vi "Upgrade Addon to Latest Version.vi"(8 "error in (no error)":errorcluster, 11 "Device Item Ref in in":T1 format="%.0x") -> (0 "error out":errorcluster, 3 "Device Item Ref out":T1 format="%.0x")   [LabVIEW 2019, in "FPGA Addon Shared.lvlib"]
uses:
  FPGA Addon Shared.lvlib
  FG Action.ctl
  Constants.vi
  Data Type.ctl
  Register Information.ctl
  <vilib>/NI/NI VeriStand Advanced SysDef API/SysDef API/Advanced System Definition.lvlib
  <vilib>/NI/NI VeriStand Advanced SysDef API/_SubVIs/SysDef.Search.GUID.vi
  <vilib>/NI/NI VeriStand Advanced SysDef API/_SubVIs/SysDef.Property.Get.Variant.vi
  <vilib>/rvi/ClientSDK/Core/ModuleGeneration/CommunicationInterfaceUtility/niFpgaDmaChannelImplementation.ctl
  <vilib>/rvi/DataTransferAndStorage/Container/Common/niFpgaDataTypeControl.ctl
  <vilib>/rvi/FIFO/Fifo_Types/Fifo_DMA_Config.ctl
  DMA Information.ctl
  NationalInstruments.VeriStand.SystemDefinitionAPI
  <vilib>/NI VeriStand/Custom Device API/Custom Device Item Ref.ctl
  <vilib>/NI VeriStand/Custom Device API/Custom Device API.lvlib
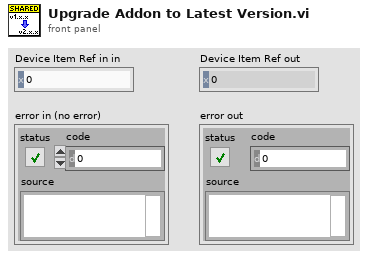
[diagram p1: front panel]
types:
  T1 = typedef "Custom Device API.lvlib/Custom Device Item Ref.ctl" = u64
  T2 = typedef "FPGA Addon Shared.lvlib/FG Action.ctl" = enum8{"GET", "SET"}
  T3 = typedef "FPGA Addon Shared.lvlib/Register Information.ctl" = cluster{"Name":string, "Data Type":T4, "Default Value":variant}
  T4 = typedef "FPGA Addon Shared.lvlib/Data Type.ctl" = enum8{"<Null>", "I8", "I16", "I32", "I64", "U8", "U16", "U32", "U64", "SGL", "Boolean", "Analog PWM In Settings", "Analog PWM In", "Digital PWM In Settings", "Digital PWM In", "Digital PWM Out", "Sine Out", "FXP+/-24.5", "FXP+/-16.5", "FXP+/-32.8", "FXP+/-64.32", "FXP+/-16.7", "FXP+/-20.5", "FXP+/-27.5", "FXP+/-32.16", "FXP +16.3", "FXP +18.3", "Digital Static In", "Digital Static Out", "Digital Static In Settings", "Digital WSS Out", "Quad Encoder Settings", "Quad Encoder In"}
  T5 = typedef "FPGA Addon Shared.lvlib/DMA Information.ctl" = cluster{"Name":string, "Data Type":T4}
  T6 = cluster{"Name":string, "Data Type":enum8{"<Null>", "I8", "I16", "I32", "I64", "U8", "U16", "U32", "U64", "SGL", "DBL", "EXT", "CSG", "CDB", "CXT", "0x0F", "0x10", "0x11", "0x12", "0x13", "0x14", "Enum U8", "Enum U16", "Enum U32", "Enum U64", "SGL PQ", "DBL PQ", "EXT PQ", "CSG PQ", "CDB PQ", "CXT PQ", "0x1F", "0x20", "Boolean", "0x22", "0x23", "0x24", "0x25", "0x26", "0x27", "0x28", "0x29", "0x2A", "0x2B", "0x2C", "0x2D", "0x2E", "0x2F", "String", "0x31", "Path", "Pict", "0x34", "0x35", "0x36", "DAQ", "0x38", "0x39", "0x3A", "0x3B", "0x3C", "0x3D", "0x3E", "0x3F", "Array", "0x41", "0x42", "0x43", "0x44", "0x45", "0x46", "0x47", "0x48", "0x49", "0x4A", "0x4B", "0x4C", "0x4D", "0x4E", "0x4F", "Cluster", "0x51", "0x52", "Variant", "Waveform", "0x55", "0x56", "0x57", "0x58", "0x59", "0x5A", "0x5B", "0x5C", "0x5D", "0x5E", "0x5F", "0x60", "0x61", "0x62", "0x63", "0x64", "0x65", "0x66", "0x67", "0x68", "0x69", "0x6A", "0x6B", "0x6C", "0x6D", "0x6E", "0x6F", "Refnum"}, "Default Value":dbl}[]
  T7 = enum8{"<Null>", "I8", "I16", "I32", "I64", "U8", "U16", "U32", "U64", "SGL", "DBL", "EXT", "CSG", "CDB", "CXT", "0x0F", "0x10", "0x11", "0x12", "0x13", "0x14", "Enum U8", "Enum U16", "Enum U32", "Enum U64", "SGL PQ", "DBL PQ", "EXT PQ", "CSG PQ", "CDB PQ", "CXT PQ", "0x1F", "0x20", "Boolean", "0x22", "0x23", "0x24", "0x25", "0x26", "0x27", "0x28", "0x29", "0x2A", "0x2B", "0x2C", "0x2D", "0x2E", "0x2F", "String", "0x31", "Path", "Pict", "0x34", "0x35", "0x36", "DAQ", "0x38", "0x39", "0x3A", "0x3B", "0x3C", "0x3D", "0x3E", "0x3F", "Array", "0x41", "0x42", "0x43", "0x44", "0x45", "0x46", "0x47", "0x48", "0x49", "0x4A", "0x4B", "0x4C", "0x4D", "0x4E", "0x4F", "Cluster", "0x51", "0x52", "Variant", "Waveform", "0x55", "0x56", "0x57", "0x58", "0x59", "0x5A", "0x5B", "0x5C", "0x5D", "0x5E", "0x5F", "0x60", "0x61", "0x62", "0x63", "0x64", "0x65", "0x66", "0x67", "0x68", "0x69", "0x6A", "0x6B", "0x6C", "0x6D", "0x6E", "0x6F", "Refnum"}
  T8 = typedef "Fifo_DMA_Config.ctl" = cluster{"Name":string, "Depth":u32, "Write? (Deprecated:Use Implementation)":bool, "Physical Channel":u32, "Base Address":u32, "Data Width":u32, "Data Type":T9, "FXP Properties":variant, "Write Window Address":u32, "Implementation":T10, "Control Set":u32}
  T9 = typedef "niFpgaDataTypeControl.ctl" = enum32{"Boolean", "I8", "I16", "I32", "I64", "U8", "U16", "U32", "U64", "FXP", "CustomControl", "SGL"}
  T10 = typedef "niFpgaDmaChannelImplementation.ctl" = enum16{"niFpgaTargetToHost", "niFpgaHostToTarget", "niFpgaPeerToPeerWriter", "niFpgaPeerToPeerReader", "niCoreTargetToHost", "niCoreHostToTarget"}
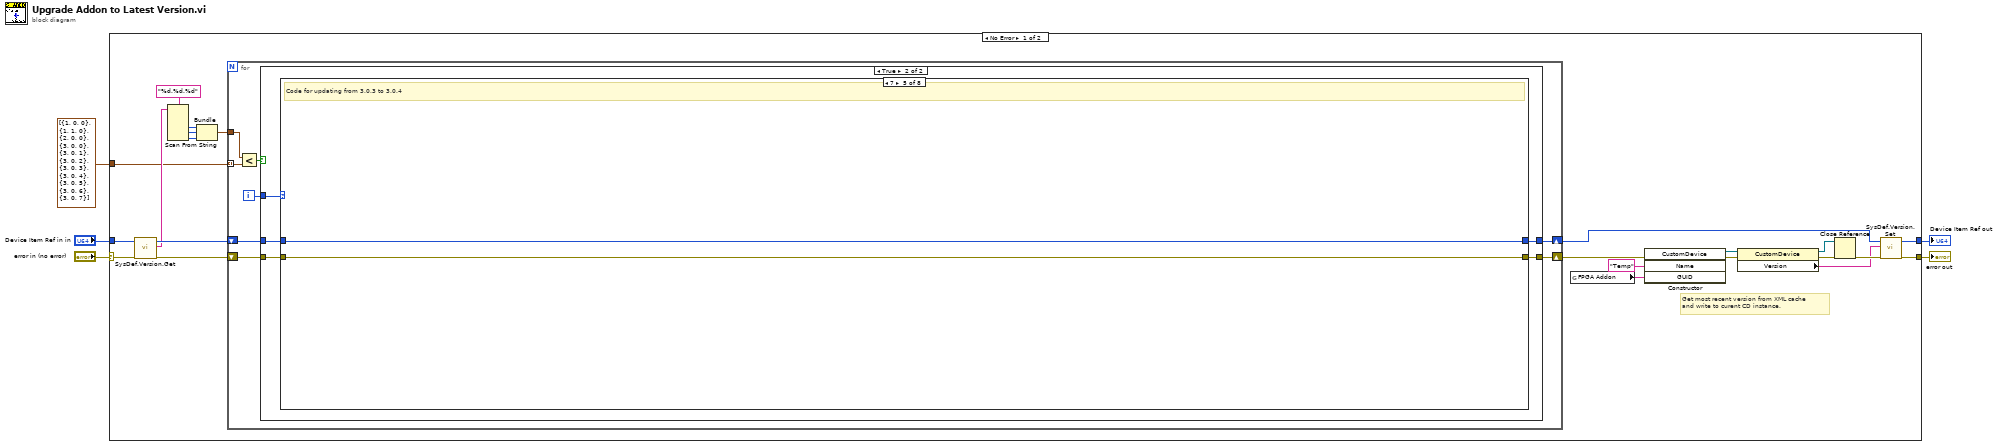
[diagram p0: block diagram]
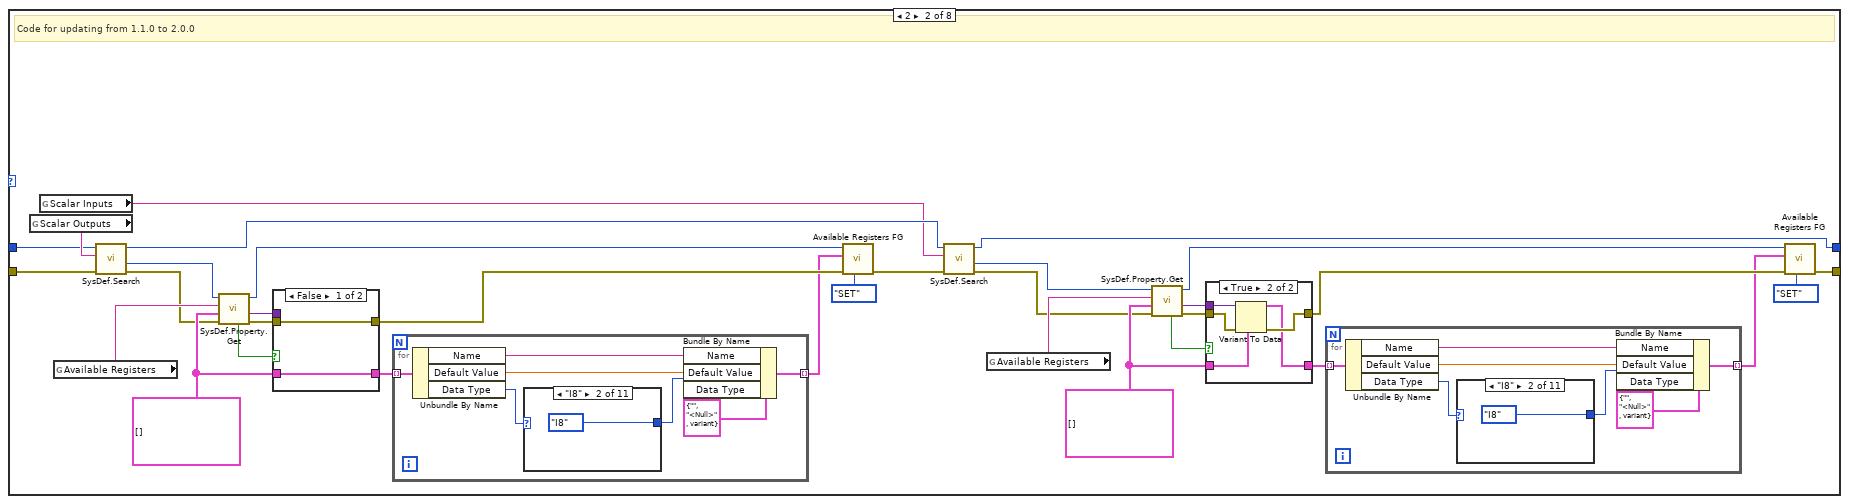
[diagram p4: hidden frame]
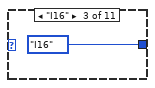
[diagram p6: hidden frame]
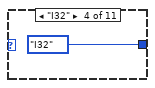
[diagram p7: hidden frame]
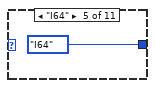
[diagram p8: hidden frame]
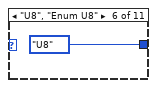
[diagram p9: hidden frame]
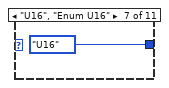
[diagram p10: hidden frame]
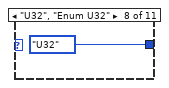
[diagram p11: hidden frame]
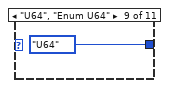
[diagram p12: hidden frame]
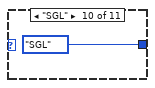
[diagram p13: hidden frame]
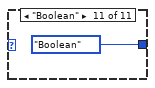
[diagram p14: hidden frame]
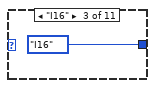
[diagram p17: hidden frame]
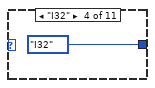
[diagram p18: hidden frame]
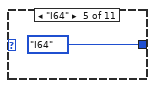
[diagram p19: hidden frame]
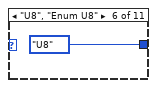
[diagram p20: hidden frame]
diagram:
  n1 = case shown="No Error" "error in (no error)" {
    selector: "error in (no error)" -> [w12 w193]
    tunnel: [w22 w193] -> w4
    tunnel: "Device Item Ref in in" -> [w11 w192]
    tunnel: [w21 w192] -> w5
    tunnel: cluster{i32, i32, i32}[] [{1, 0, 0}, {1, 1, 0}, {2, 0, 0}, {3, 0, 0}, {3, 0, 1}, {3, 0, 2}, {3, 0, 3}, {3, 0, 4}, {3, 0, 5}, {3, 0, 6}, {3, 0, 7}] -> [w6 _]
    frame No Error {
      # "Get most recent version from XML cache\nand write to curent CD instance."
      n2 = call <vilib>:"SysDef.Version.Get.vi"("error in (no error)"=w12, "nodeID"=w11) -> ("error out"=w9:errorcluster, "Version"=w8:string, "nodeID out"=w10:u64)  [unwired: 7 in]
      n3 = Scan From String(format string="%d.%d.%d", input string=w8) -> (output 1=w15:i32, output 2=w14:i32, output 3=w16:i32)  [unwired: 5 in, 3 out]
      n4 = Bundle(w15, w14, w16) -> (w7:cluster{i32, i32, i32})  [unwired: 1 in]
      n5 = for {
        shift-right: [w36] -> w19
        shift-left: w9 -> [w29]
        shift-right: [w35] -> w20
        shift-left: w10 -> [w30]
        tunnel: w7 -> [w33]
        tunnel: w6 -> [w31] mode=indexing
        i -> [w34]
        n6 = Less?(x=w33, y=w31) -> (x < y?=w32:bool)
        n7 = case shown="True" w32 {
          tunnel: w29 -> [w38 w43]
          tunnel: [w38 w42] -> w36
          tunnel: w30 -> [w37 w39]
          tunnel: [w37 w40] -> w35
          tunnel: w34 -> [_ w41]
          frame False {
          }
          frame True {
            n8 = case shown="7" w41 {
              tunnel: w43 -> [w45 w71 w151 w183 w185 w187 w189 w191]
              tunnel: [w45 w46 w127 w183 w185 w187 w189 w191] -> w42
              tunnel: [w44 w47 w128 w182 w184 w186 w188 w190] -> w40
              tunnel: w39 -> [w44 w70 w150 w182 w184 w186 w188 w190]
              frame Default {
              }
              frame 2 {
                w54 = T6 [] ("Available Registers 2")
                w65 = T6 [] ("Available Registers 2")
                # "Code for updating from 1.1.0 to 2.0.0"
                n9 = global read "Constants.vi" "Scalar Outputs"() -> (w76:string)
                n10 = global read "Constants.vi" "Scalar Inputs"() -> (w72:string)
                n11 = global read "Constants.vi" "Available Registers"() -> (w66:string)
                n12 = call-poly <vilib>:"SysDef.Search.vi"("error in (no error)"=w71, "GUID"=w76, "nodeID"=w70) -> ("error out"=w62:errorcluster, "Value out"=w64:u64, "nodeID out"=w73:u64)  [unwired: 5 in, 1 out]
                n13 = call-poly <vilib>:"SysDef.Property.Get.vi"("error in (no error)"=w62, "Value"=w65, "Property Name"=w66, "nodeID"=w64) -> ("error out"=w68:errorcluster, "Value"=w67:variant, "nodeID out"=w63:u64, "Found?"=w69:bool)  [unwired: 4 in]
                n14 = case shown="False" w69 {
                  tunnel: w67 -> [_ w125]
                  tunnel: w65 -> [w119 w124]
                  tunnel: w68 -> [w120 w123]
                  tunnel: [w120 w122] -> w61
                  tunnel: [w119 w121] -> w60
                  frame False {
                  }
                  frame True {
                    n15 = Variant To Data(error in=w123, type=w124, Variant=w125) -> (data=w121:T6, error out=w122:errorcluster)
                  }
                }
                n16 = for {
                  tunnel: w60 -> [w108] mode=indexing
                  tunnel: [w104] -> w59 mode=indexing
                  n17 = Unbundle By Name(w108) -> ("Name"=w107:string, "Default Value"=w106:dbl, "Data Type"=w103:T7)
                  n18 = case shown="\"I8\"" w103 {
                    tunnel: [_ Data_Type."I8" ("Data Type") Data_Type."I16" ("Data Type") Data_Type."I32" ("Data Type") Data_Type."I64" ("Data Type") Data_Type."U8" ("Data Type") Data_Type."U16" ("Data Type") Data_Type."U32" ("Data Type") Data_Type."U64" ("Data Type") Data_Type."SGL" ("Data Type") Data_Type."Boolean" ("Data Type")] -> w102
                    frame Default {
                    }
                    frame "I8" {
                    }
                    frame "I16" {
                    }
                    frame "I32" {
                    }
                    frame "I64" {
                    }
                    frame "U8", "Enum U8" {
                    }
                    frame "U16", "Enum U16" {
                    }
                    frame "U32", "Enum U32" {
                    }
                    frame "U64", "Enum U64" {
                    }
                    frame "SGL" {
                    }
                    frame "Boolean" {
                    }
                  }
                  n19 = Bundle By Name(cluster=T3 {"Name"="", "Data Type"=enum."<Null>", "Default Value"=variant(refnum<class> refnum)}, "Name"=w107, "Default Value"=w106, "Data Type"=w102) -> (w104:T3)
                }
                n20 = call "Available Registers FG.vi"("Action"=FG_Action."SET", "error in (no error)"=w61, "Available Registers"=w59, "Item Ref"=w63) -> ("error out"=w74:errorcluster)  [unwired: 5 in, 2 out]
                n21 = call-poly <vilib>:"SysDef.Search.vi"("error in (no error)"=w74, "GUID"=w72, "nodeID"=w73) -> ("error out"=w52:errorcluster, "Value out"=w49:u64, "nodeID out"=w47:u64)  [unwired: 5 in, 1 out]
                n22 = global read "Constants.vi" "Available Registers"() -> (w55:string)
                n23 = call-poly <vilib>:"SysDef.Property.Get.vi"("error in (no error)"=w52, "Value"=w54, "Property Name"=w55, "nodeID"=w49) -> ("error out"=w57:errorcluster, "Value"=w56:variant, "nodeID out"=w48:u64, "Found?"=w58:bool)  [unwired: 4 in]
                n24 = case shown="True" w58 {
                  tunnel: w56 -> [_ w101]
                  tunnel: w54 -> [w95 w100]
                  tunnel: w57 -> [w96 w99]
                  tunnel: [w96 w98] -> w51
                  tunnel: [w95 w97] -> w53
                  frame False {
                  }
                  frame True {
                    n25 = Variant To Data(error in=w99, type=w100, Variant=w101) -> (data=w97:T6, error out=w98:errorcluster)
                  }
                }
                n26 = for {
                  tunnel: w53 -> [w84] mode=indexing
                  tunnel: [w80] -> w50 mode=indexing
                  n27 = Unbundle By Name(w84) -> ("Name"=w83:string, "Default Value"=w82:dbl, "Data Type"=w79:T7)
                  n28 = case shown="\"I8\"" w79 {
                    tunnel: [_ Data_Type."I8" ("Data Type") Data_Type."I16" ("Data Type") Data_Type."I32" ("Data Type") Data_Type."I64" ("Data Type") Data_Type."U8" ("Data Type") Data_Type."U16" ("Data Type") Data_Type."U32" ("Data Type") Data_Type."U64" ("Data Type") Data_Type."SGL" ("Data Type") Data_Type."Boolean" ("Data Type")] -> w78
                    frame Default {
                    }
                    frame "I8" {
                    }
                    frame "I16" {
                    }
                    frame "I32" {
                    }
                    frame "I64" {
                    }
                    frame "U8", "Enum U8" {
                    }
                    frame "U16", "Enum U16" {
                    }
                    frame "U32", "Enum U32" {
                    }
                    frame "U64", "Enum U64" {
                    }
                    frame "SGL" {
                    }
                    frame "Boolean" {
                    }
                  }
                  n29 = Bundle By Name(cluster=T3 {"Name"="", "Data Type"=enum."<Null>", "Default Value"=variant(refnum<class> refnum)}, "Name"=w83, "Default Value"=w82, "Data Type"=w78) -> (w80:T3)
                }
                n30 = call "Available Registers FG.vi"("Action"=FG_Action."SET", "error in (no error)"=w51, "Available Registers"=w50, "Item Ref"=w48) -> ("error out"=w46:errorcluster)  [unwired: 5 in, 2 out]
              }
              frame 5 {
                w126 = T8[] [] ("Available Registers 2")
                w135 = T8[] [] ("Available Registers 2")
                # "Code for updating from 3.0.1 to 3.0.2"
                n31 = global read "Constants.vi" "Waveform Outputs"() -> (w152:string)
                n32 = global read "Constants.vi" "Waveform Inputs"() -> (w156:string)
                n33 = global read "Constants.vi" "Available DMA"() -> (w146:string)
                n34 = call-poly <vilib>:"SysDef.Search.vi"("error in (no error)"=w151, "GUID"=w156, "nodeID"=w150) -> ("error out"=w143:errorcluster, "Value out"=w145:u64, "nodeID out"=w153:u64)  [unwired: 5 in, 1 out]
                n35 = call-poly <vilib>:"SysDef.Property.Get.vi"("error in (no error)"=w143, "Value"=w126, "Property Name"=w146, "nodeID"=w145) -> ("error out"=w148:errorcluster, "Value"=w147:variant, "nodeID out"=w144:u64, "Found?"=w149:bool)  [unwired: 4 in]
                n36 = case shown="False" w149 {
                  tunnel: w147 -> [_ w181]
                  tunnel: w126 -> [w175 w180]
                  tunnel: w148 -> [w176 w179]
                  tunnel: [w176 w178] -> w142
                  tunnel: [w175 w177] -> w141
                  frame False {
                  }
                  frame True {
                    n37 = Variant To Data(error in=w179, type=w180, Variant=w181) -> (data=w177:T8[], error out=w178:errorcluster)
                  }
                }
                n38 = for {
                  tunnel: w141 -> [w174] mode=indexing
                  tunnel: [w172] -> w140 mode=indexing
                  n39 = Unbundle By Name(w174) -> ("Name"=w173:string)
                  n40 = Bundle By Name(cluster=T5 {"Name"="", "Data Type"=enum."<Null>"} ("Cluster"), "Name"=w173, "Data Type"=Data_Type."SGL") -> (w172:T5)
                }
                n41 = call "Available DMA FG.vi"("Action"=FG_Action."SET", "error in (no error)"=w142, "Available DMA"=w140, "Item Ref"=w144) -> ("error out"=w154:errorcluster)  [unwired: 5 in, 2 out]
                n42 = call-poly <vilib>:"SysDef.Search.vi"("error in (no error)"=w154, "GUID"=w152, "nodeID"=w153) -> ("error out"=w133:errorcluster, "Value out"=w130:u64, "nodeID out"=w128:u64)  [unwired: 5 in, 1 out]
                n43 = global read "Constants.vi" "Available DMA"() -> (w136:string)
                n44 = call-poly <vilib>:"SysDef.Property.Get.vi"("error in (no error)"=w133, "Value"=w135, "Property Name"=w136, "nodeID"=w130) -> ("error out"=w138:errorcluster, "Value"=w137:variant, "nodeID out"=w129:u64, "Found?"=w139:bool)  [unwired: 4 in]
                n45 = case shown="False" w139 {
                  tunnel: w137 -> [_ w169]
                  tunnel: w135 -> [w163 w168]
                  tunnel: w138 -> [w164 w167]
                  tunnel: [w164 w166] -> w132
                  tunnel: [w163 w165] -> w134
                  frame False {
                  }
                  frame True {
                    n46 = Variant To Data(error in=w167, type=w168, Variant=w169) -> (data=w165:T8[], error out=w166:errorcluster)
                  }
                }
                n47 = for {
                  tunnel: w134 -> [w162] mode=indexing
                  tunnel: [w160] -> w131 mode=indexing
                  n48 = Unbundle By Name(w162) -> ("Name"=w161:string)
                  n49 = Bundle By Name(cluster=T5 {"Name"="", "Data Type"=enum."<Null>"} ("Cluster"), "Name"=w161, "Data Type"=Data_Type."SGL") -> (w160:T5)
                }
                n50 = call "Available DMA FG.vi"("Action"=FG_Action."SET", "error in (no error)"=w132, "Available DMA"=w131, "Item Ref"=w129) -> ("error out"=w127:errorcluster)  [unwired: 5 in, 2 out]
              }
              frame 6 {
                # "Code for updating from 3.0.2 to 3.0.3"
              }
              frame 7 {
                # "Code for updating from 3.0.3 to 3.0.4"
              }
              frame 8 {
                # "Code for updating from 3.0.4 to 3.0.5"
              }
              frame 9 {
                # "Code for updating from 3.0.5 to 3.0.6"
              }
              frame 10 {
                # "Code for updating from 3.0.6 to 3.0.7"
              }
            }
          }
        }
      }
      n51 = global read "Constants.vi" "FPGA Addon"() -> (w17:string)
      n52 = constructor class="CustomDevice"(error in=w19, "Name"="Temp", "GUID"=w17) -> (reference out=w28:refnum<k24>, error out=w27:errorcluster)  [unwired: 2 in, 3 out]
      n53 = property class="CustomDevice"(reference=w28, error in=w27) -> (reference out=w25:refnum<k24>, error out=w26:errorcluster, "Version"=w23:string)
      n54 = Close Reference(reference=w25, error in (no error)=w26) -> (error out=w24:errorcluster)
      n55 = call <vilib>:"SysDef.Version.Set.vi"("error in (no error)"=w24, "Version"=w23, "nodeID"=w20) -> ("error out"=w22:errorcluster, "nodeID out"=w21:u64)  [unwired: 7 in]
    }
    frame Error {
    }
  }
  "Device Item Ref out" <- w5
  "error out" <- w4
